vi "Destroy User Events.vi"(11 "UI Template in":refnum<class "Generador funciones ACQ.lvclass">) -> (3 "UI Template out":refnum<class "Generador funciones ACQ.lvclass">)   [LabVIEW 2019, in "Generador funciones ACQ.lvlib" / "Generador funciones ACQ.lvclass"]
uses:
  Generador funciones ACQ.lvclass
  Generador funciones ACQ.lvclass/Generador funciones ACQ.ctl
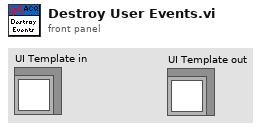
[diagram p1: front panel]
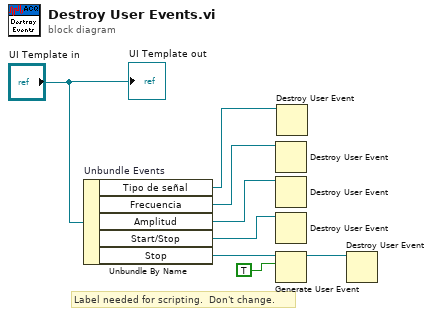
[diagram p0: block diagram]
diagram:
  # "Label needed for scripting.  Don't change."
  n1 = Unbundle By Name "Unbundle Events"("UI Template in") -> ("Tipo de señal"=w1:refnum<user-event>, "Frecuencia"=w4:refnum<user-event>, "Amplitud"=w3:refnum<user-event>, "Start/Stop"=w2:refnum<user-event>, "Stop"=w6:refnum<user-event>)
  n2 = Destroy User Event(user event=w4) -> ()  [unwired: 1 in, 1 out]
  n3 = Destroy User Event(user event=w3) -> ()  [unwired: 1 in, 1 out]
  n4 = Destroy User Event(user event=w2) -> ()  [unwired: 1 in, 1 out]
  n5 = Generate User Event(user event=w6, event data cluster=TRUE ("event data")) -> (user event out=w7:refnum<user-event>)  [unwired: 2 in, 1 out]
  n6 = Destroy User Event(user event=w1) -> ()  [unwired: 1 in, 1 out]
  n7 = Destroy User Event(user event=w7) -> ()  [unwired: 1 in, 1 out]
  "UI Template out" <- "UI Template in"
